vi "Write Motor Controller Names.vi"(8 "error in (no error)":errorcluster, 10 "Motor Controller Names":T1, 11 "Tank Drive in":refnum<class "Tank Drive.lvclass">) -> (0 "error out":errorcluster, 3 "Tank Drive out":refnum<class "Tank Drive.lvclass">)   [LabVIEW 2019, in "Drive.lvlib" / "Tank Drive.lvclass"]
uses:
  Tank Drive.lvclass
  Controls/Motor Controller Names.ctl
  Tank Drive.lvclass/Tank Drive.ctl
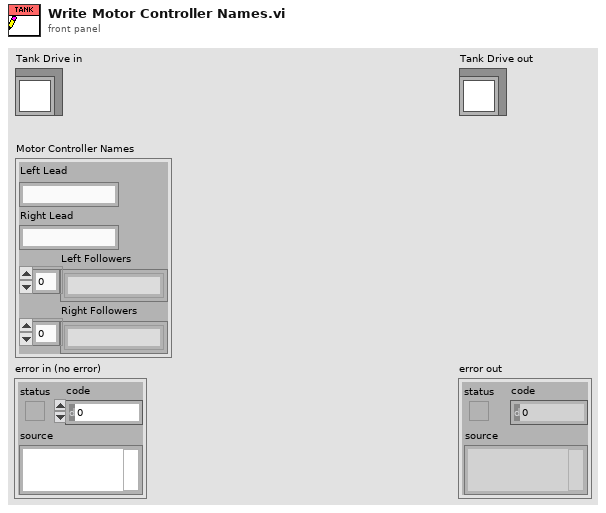
[diagram p1: front panel]
types:
  T1 = typedef "Drive.lvlib/Tank Drive.lvclass/Motor Controller Names.ctl" = cluster{"Left Lead":string, "Right Lead":string, "Left Followers":string[], "Right Followers":string[]}
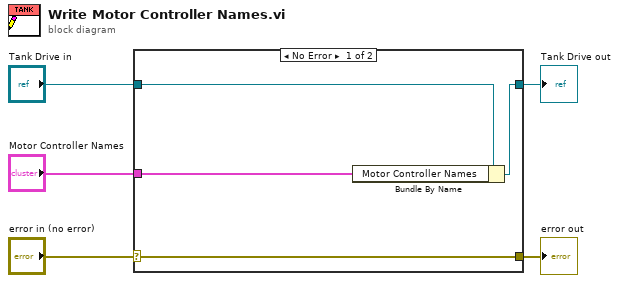
[diagram p0: block diagram]
diagram:
  n1 = case shown="No Error" "error in (no error)" {
    selector: "error in (no error)" -> [w9 w10]
    tunnel: [w9 w10] -> w4
    tunnel: [w7 w11] -> w2
    tunnel: "Tank Drive in" -> [w8 w11]
    tunnel: "Motor Controller Names" -> [w6 _]
    frame No Error {
      n2 = Bundle By Name(cluster=w8, "Motor Controller Names"=w6) -> (w7:refnum<class "Tank Drive.lvclass">)
    }
    frame Error {
    }
  }
  "error out" <- w4
  "Tank Drive out" <- w2
